vi "Determine Warning State Machine.vi"(6 "최대 풍속":dbl, 7 "현재 풍속":dbl, 9 "최저 온도":dbl, 10 "최고 온도":dbl, 11 "현재 온도":dbl) -> (1 "경고?":bool, 2 "경고 텍스트":string)   [LabVIEW 2010]
doc: "이 VI는 LabVIEW Core II의 연습문제로서 사용되는 상속된 코드의 확장 가능하고 관리하기 쉽고 읽기 쉬운 버전입니다."
uses:
  Det Warnings.ctl
panel:
  out "에러 출력":cluster{"상태":bool, "코드":i32, "소스":string}
  in  "에러 입력(에러 없음)":cluster{"상태":bool, "코드":i32, "소스":string}
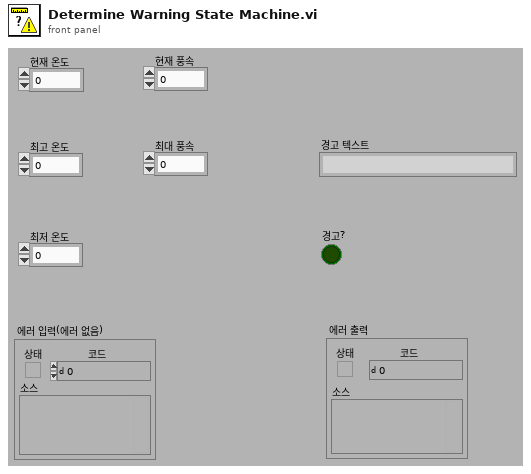
[diagram p1: front panel]
types:
  T1 = typedef "Det Warnings.ctl" = enum16{"열사병", "동상", "강풍", "경고 생성"}
  T2 = cluster{"현재 온도":dbl, "최고 온도":dbl, "최저 온도":dbl, "현재 풍속":dbl, "최대 풍속":dbl}
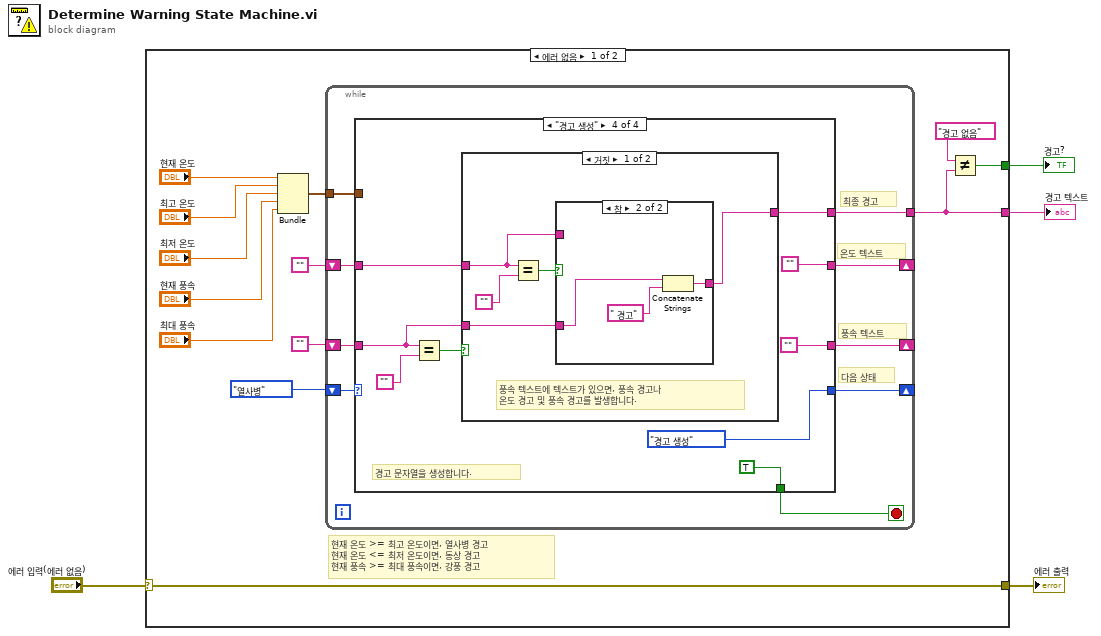
[diagram p0: block diagram]
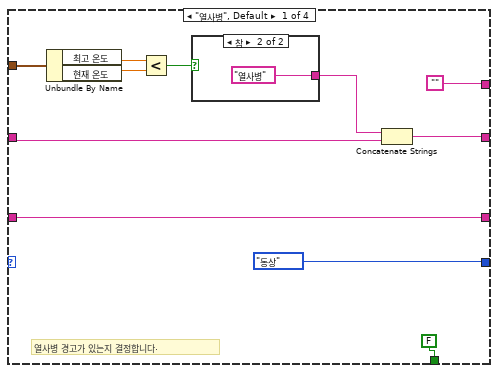
[diagram p2: hidden frame]
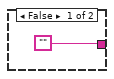
[diagram p3: hidden frame]
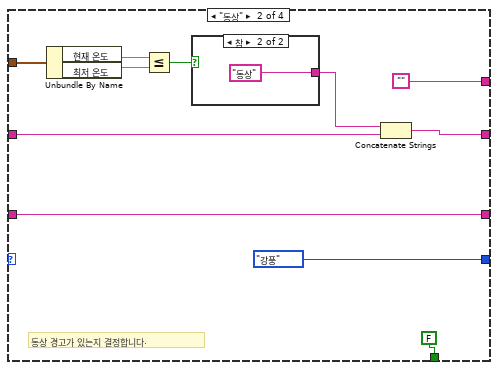
[diagram p4: hidden frame]
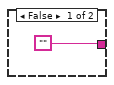
[diagram p5: hidden frame]
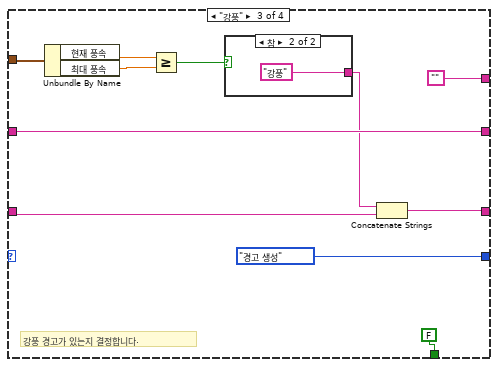
[diagram p6: hidden frame]
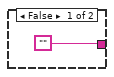
[diagram p7: hidden frame]
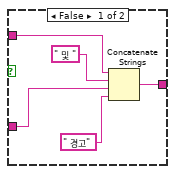
[diagram p8: hidden frame]
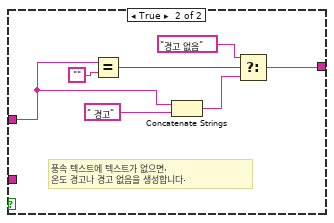
[diagram p9: hidden frame]
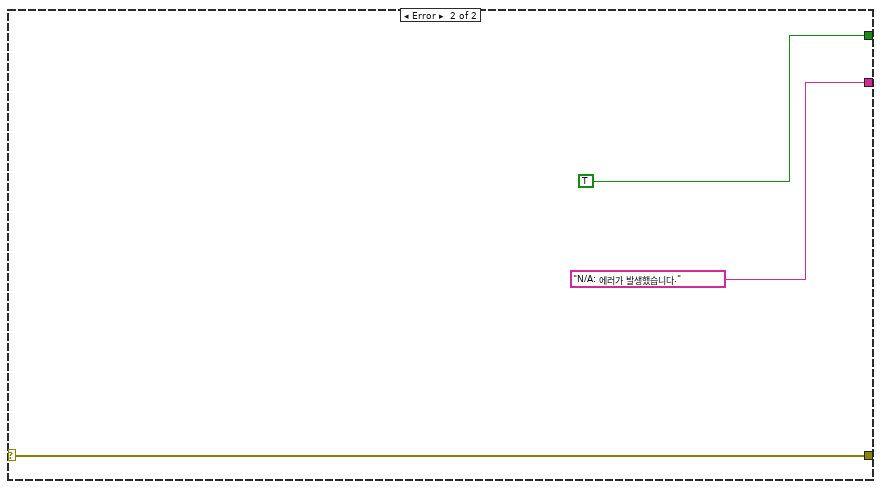
[diagram p10: hidden frame]
diagram:
  n1 = case shown="에러 없음" "에러 입력(에러 없음)" {
    selector: "에러 입력(에러 없음)" -> [w16 w97]
    tunnel: [w16 w97] -> w1
    tunnel: [w17 TRUE] -> w4
    tunnel: [w6 "N/A: 에러가 발생했습니다." ("f")] -> w3
    frame No Error {
      # "현재 온도 >= 최고 온도이면, 열사병 경고\n현재 온도 <= 최저 온도이면, 동상 경고\n현재 풍속 >= 최대 풍속이면, 강풍 경고"
      n2 = Bundle("현재 온도"="현재 온도", "최고 온도"="최고 온도", "최저 온도"="최저 온도", "현재 풍속"="현재 풍속", "최대 풍속"="최대 풍속") -> (w9:T2)  [unwired: 1 in]
      n3 = while {
        tunnel: w9 -> [w23]
        shift-right: [w22] -> _
        shift-left: Det_Warnings."열사병" ("Enum") -> [w26]
        shift-right: [w25] -> _
        shift-left: "" -> [w21]
        shift-right: [w24] -> _
        shift-left: "" -> [w20]
        tunnel: [w19] -> w6
        stop <- w18 stop-if-true
        # "최종 경고"
        # "다음 상태"
        # "풍속 텍스트"
        # "온도 텍스트"
        n4 = case shown="\"경고 생성\"" w26 {
          tunnel: [w29 w45 w57 ""] -> w24
          tunnel: [w32 w44 w58 ""] -> w25
          tunnel: w23 -> [w36 w50 w63 _]
          tunnel: [Det_Warnings."동상" ("Enum") Det_Warnings."강풍" ("Enum") Det_Warnings."경고 생성" ("Enum") Det_Warnings."경고 생성" ("Enum")] -> w22
          tunnel: w21 -> [w31 w42 w58 w74]
          tunnel: w20 -> [w29 w45 w55 w71]
          tunnel: ["" "" "" w70] -> w19
          tunnel: [FALSE FALSE FALSE TRUE] -> w18
          frame "열사병", Default {
            # "열사병 경고가 있는지 결정합니다."
            n5 = Unbundle By Name(w36) -> ("최고 온도"=w35:dbl, "현재 온도"=w34:dbl)
            n6 = Less?(x=w35, y=w34) -> (x < y?=w37:bool)
            n7 = case shown="참" w37 {
              tunnel: ["" "열사병"] -> w30
              frame False {
              }
              frame True {
              }
            }
            n8 = Concatenate Strings(w30, w31) -> (w32:string)
          }
          frame "동상" {
            # "동상 경고가 있는지 결정합니다."
            n9 = Unbundle By Name(w50) -> ("현재 온도"=w48:dbl, "최저 온도"=w47:dbl)
            n10 = Less Or Equal?(x=w48, y=w47) -> (x <= y?=w49:bool)
            n11 = case shown="참" w49 {
              tunnel: ["" "동상"] -> w43
              frame False {
              }
              frame True {
              }
            }
            n12 = Concatenate Strings(w43, w42) -> (w44:string)
          }
          frame "강풍" {
            # "강풍 경고가 있는지 결정합니다."
            n13 = Unbundle By Name(w63) -> ("현재 풍속"=w62:dbl, "최대 풍속"=w61:dbl)
            n14 = Greater Or Equal?(x=w62, y=w61) -> (x >= y?=w60:bool)
            n15 = case shown="참" w60 {
              tunnel: ["" "강풍"] -> w56
              frame False {
              }
              frame True {
              }
            }
            n16 = Concatenate Strings(w56, w55) -> (w57:string)
          }
          frame "경고 생성" {
            # "경고 문자열을 생성합니다."
            n17 = Equal?(x=w71, y="") -> (x = y?=w72:bool)
            n18 = case shown="거짓" w72 {
              tunnel: [w77 w89] -> w70
              tunnel: w74 -> [w75 w93]
              tunnel: w71 -> [w76 _]
              frame False {
                # "풍속 텍스트에 텍스트가 있으면, 풍속 경고나 \n온도 경고 및 풍속 경고를 발생합니다."
                n19 = Equal?(x=w75, y="") -> (x = y?=w78:bool)
                n20 = case shown="참" w78 {
                  tunnel: [w82 w86] -> w77
                  tunnel: w76 -> [w81 w85]
                  tunnel: w75 -> [w80 _]
                  frame False {
                    n21 = Concatenate Strings(w80, " 및 " ("string"), w81, " 경고" ("string")) -> (w82:string)
                  }
                  frame True {
                    n22 = Concatenate Strings(w85, " 경고" ("string")) -> (w86:string)
                  }
                }
              }
              frame True {
                # "풍속 텍스트에 텍스트가 없으면, \n온도 경고나 경고 없음을 생성합니다."
                n23 = Equal?(x=w93, y="") -> (x = y?=w92:bool)
                n24 = Concatenate Strings(w93, " 경고") -> (w88:string)
                n25 = Select(t="경고 없음" ("string"), s=w92, f=w88) -> (s? t:f=w89:string)
              }
            }
          }
        }
      }
      n26 = Not Equal?(x="경고 없음", y=w6) -> (x != y?=w17:bool)
    }
    frame Error {
    }
  }
  "경고 텍스트" <- w3
  "경고?" <- w4
  "에러 출력" <- w1
